vi "PLC指令转换.vi"(11 "PLC指令":T1={"变量类型"=2, "PLC地址"=0, "size"=0, "写入数据(写入时有效)"=0} {"变量类型" items=["X", "Y", "M", "D"]}) -> (1 "IpsData":i16, 2 "size":i32, 3 "szDeviceList":string)   [LabVIEW 2015, in "Action.lvlib"]
uses:
  Action.lvlib
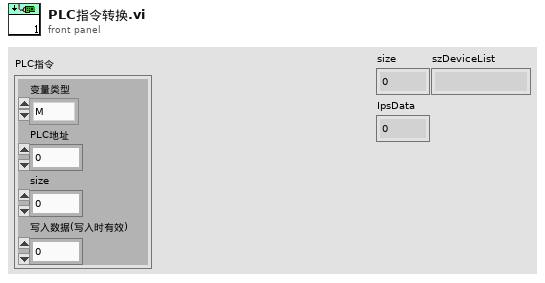
[diagram p1: front panel]
types:
  T1 = typedef "Action.lvlib/PLC控制指令.ctl" = cluster{"变量类型":u32, "PLC地址":i32, "size":i32, "写入数据(写入时有效)":i16}
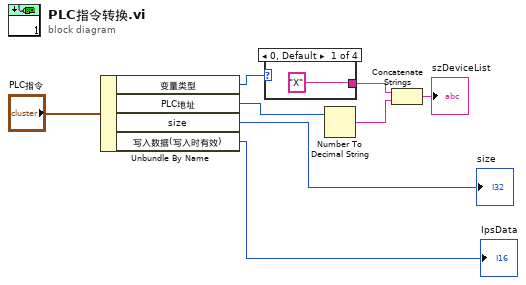
[diagram p0: block diagram]
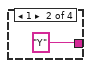
[diagram p2: hidden frame]
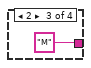
[diagram p3: hidden frame]
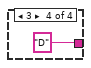
[diagram p4: hidden frame]
diagram:
  n1 = Unbundle By Name("PLC指令") -> ("变量类型"=w8:u32, "PLC地址"=w7:i32, "size"=→"size":i32, "写入数据(写入时有效)"=→"IpsData":i16)
  n2 = case shown="0, Default" w8 {
    tunnel: ["X" "Y" "M" "D"] -> w5
    frame 0, Default {
    }
    frame 1 {
    }
    frame 2 {
    }
    frame 3 {
    }
  }
  n3 = Number To Decimal String(number=w7) -> (decimal integer string=w6:string)  [unwired: 1 in]
  n4 = Concatenate Strings(w5, w6) -> (→"szDeviceList":string)
